vi "PISetAxisPosDigital.vi"(0 "Position":sgl format="%.2f", 1 "Axis":i32) -> ()   [LabVIEW 2009]
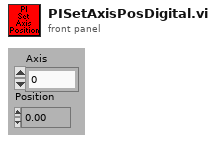
[diagram p1: front panel]
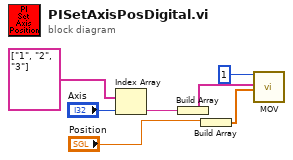
[diagram p0: block diagram]
diagram:
  n1 = Index Array(array=string[] ["1", "2", "3"], index="Axis") -> (element=w3:string)
  n2 = Build Array(w3) -> (w1:string[])
  n3 = Build Array("Position") -> (w6:sgl[])
  n4 = call "MOV.vi"("System no."=1, "Axes to move"=w1, "Position values"=w6) -> ()  [unwired: 16 in, 1 out]
